vi "Beams_Alignment.vi"() -> (3 "Boolean":bool)   [LabVIEW 2018]
panel:
  in  "Yes":bool
  in  "No":bool
  # "Can Laser Beam enter the sphere?"
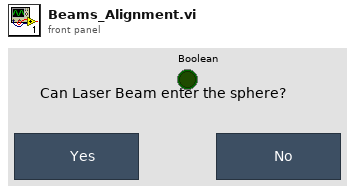
[diagram p1: front panel]
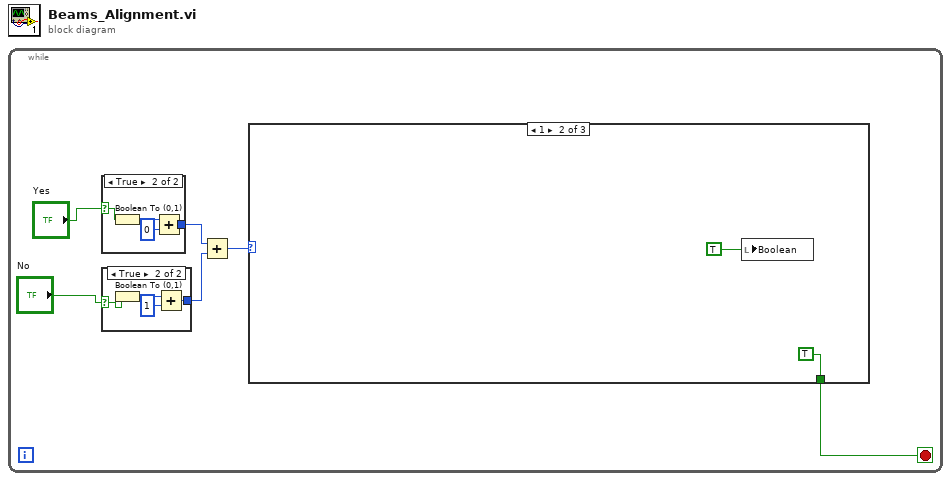
[diagram p0: block diagram]
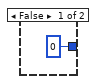
[diagram p2: hidden frame]
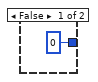
[diagram p3: hidden frame]
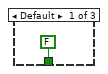
[diagram p4: hidden frame]
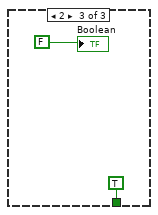
[diagram p5: hidden frame]
diagram:
  n1 = while {
    stop <- w3 stop-if-true
    n2 = case shown="True" "Yes" {
      selector: "Yes" -> [_ w8]
      tunnel: [i16 0 w9] -> w5
      frame False {
      }
      frame True {
        n3 = Boolean To (0,1)(Boolean=w8) -> (0, 1=w11:i16)
        n4 = Add(x=w11, y=i16 0) -> (x+y=w9:i16)
      }
    }
    n5 = case shown="True" "No" {
      selector: "No" -> [_ w13]
      tunnel: [i16 0 w14] -> w4
      frame False {
      }
      frame True {
        n6 = Boolean To (0,1)(Boolean=w13) -> (0, 1=w16:i16)
        n7 = Add(x=w16, y=i16 1) -> (x+y=w14:i16)
      }
    }
    n8 = Add(x=w5, y=w4) -> (x+y=w6:i16)
    n9 = case shown="1" w6 {
      tunnel: [FALSE TRUE TRUE] -> w3
      frame Default {
      }
      frame 1 {
        n10 = local write "Boolean"(TRUE) -> ()
      }
      frame 2 {
        "Boolean" <- FALSE
      }
    }
  }
